vi "qp_minMaxInfScale.vi"(7 "Xmax":dbl[](array[numeric]), 8 "Xmin":dbl[](array[numeric])) -> (0 "Xmax scale":dbl[](array[numeric]), 1 "Xmin scale":dbl[](array[numeric]), 2 "Xmax":dbl[](array[numeric]), 3 "Xmin":dbl[](array[numeric]), 4 "loop?":bool)   [LabVIEW 2020, in "NI_Gmath.lvlib"]
uses:
  NI_Gmath.lvlib
panel:
  in  "scale factor":dbl=10.0
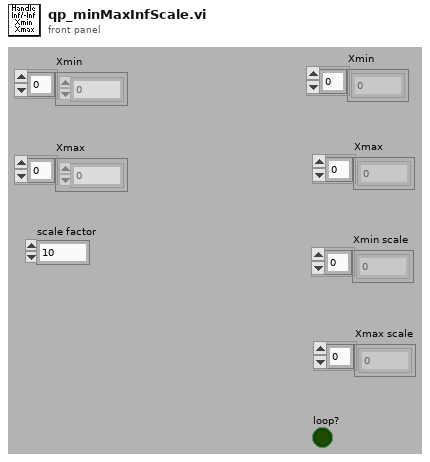
[diagram p1: front panel]
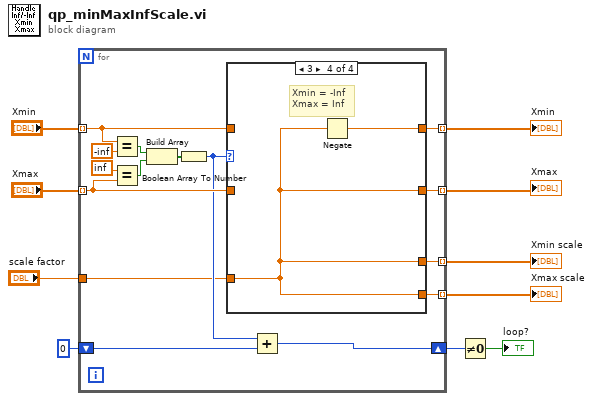
[diagram p0: block diagram]
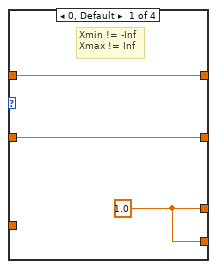
[diagram p2: hidden frame]
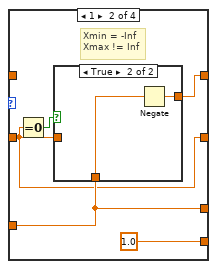
[diagram p3: hidden frame]
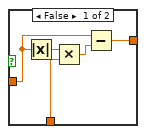
[diagram p4: hidden frame]
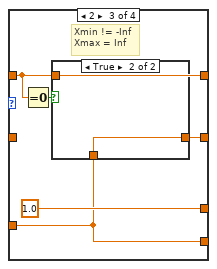
[diagram p5: hidden frame]
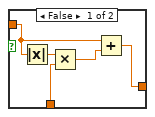
[diagram p6: hidden frame]
diagram:
  n1 = for {
    tunnel: "Xmin" -> [w19] mode=indexing
    tunnel: "Xmax" -> [w20] mode=indexing
    tunnel: [w18] -> w6 mode=indexing
    tunnel: [w17] -> w8 mode=indexing
    tunnel: [w16] -> w7 mode=indexing
    tunnel: [w15] -> w5 mode=indexing
    shift-right: [w12] -> w3
    shift-left: u32 0 -> [w13]
    tunnel: "scale factor" -> [w11]
    n2 = Equal?(x=w19, y=-inf) -> (x = y?=w24:bool)
    n3 = Equal?(x=inf, y=w20) -> (x = y?=w23:bool)
    n4 = Build Array(w24, w23) -> (w22:bool[])
    n5 = Boolean Array To Number(Boolean array=w22) -> (number=w14:u32)
    n6 = case shown="3" w14 {
      tunnel: w20 -> [w27 w30 _ _]
      tunnel: w19 -> [w28 _ w42 _]
      tunnel: [w28 w32 w42 w52] -> w17
      tunnel: [w27 w30 w44 w53] -> w16
      tunnel: [w26 w31 1.0 w53] -> w18
      tunnel: [w26 1.0 w43 w53] -> w15
      tunnel: w11 -> [_ w31 w43 w53]
      frame 0, Default {
        w26 = 1.0
        # "Xmin != -Inf\nXmax != Inf"
      }
      frame 1 {
        # "Xmin = -Inf\nXmax != Inf"
        n7 = Equal To 0?(x=w30) -> (x = 0?=w29:bool)
        n8 = case shown="True" w29 {
          tunnel: [w36 w40] -> w32
          tunnel: w30 -> [w35 _]
          tunnel: w31 -> [w34 w39]
          frame False {
            n9 = Absolute Value(x=w35) -> (abs(x)=w38:dbl)
            n10 = Multiply(x=w38, y=w34) -> (x*y=w37:dbl)
            n11 = Subtract(x=w35, y=w37) -> (x-y=w36:dbl)
          }
          frame True {
            n12 = Negate(x=w39) -> (-x=w40:dbl)
          }
        }
      }
      frame 2 {
        # "Xmin != -Inf\nXmax = Inf"
        n13 = Equal To 0?(x=w42) -> (x = 0?=w41:bool)
        n14 = case shown="True" w41 {
          tunnel: [w48 w51] -> w44
          tunnel: w42 -> [w47 _]
          tunnel: w43 -> [w46 w51]
          frame False {
            n15 = Absolute Value(x=w47) -> (abs(x)=w50:dbl)
            n16 = Multiply(x=w50, y=w46) -> (x*y=w49:dbl)
            n17 = Add(x=w47, y=w49) -> (x+y=w48:dbl)
          }
          frame True {
          }
        }
      }
      frame 3 {
        # "Xmin = -Inf\nXmax = Inf"
        n18 = Negate(x=w53) -> (-x=w52:dbl)
      }
    }
    n19 = Add(x=w14, y=w13) -> (x+y=w12:u32)
  }
  "Xmin" <- w8
  "Xmax" <- w7
  "Xmin scale" <- w6
  "Xmax scale" <- w5
  n20 = Not Equal To 0?(x=w3) -> (x != 0?=→"loop?":bool)
